vi "Process.vi"(8 "error in":errorcluster, 11 "UI_Scope":refnum<class "UI_Scope.lvclass">) -> (0 "error out":errorcluster, 3 "UI_Scope out":refnum<class "UI_Scope.lvclass">)   [LabVIEW 2016, in "UI_Scope.lvclass"]
doc: "---------------------------------------------------------------\nJKI State Machine Objects™\nhttp://jki.net/state-machine-objects/\nCopyright (C) 2005-2015, JKI <info@jki.net>\nALL RIGHTS RESERVED"
uses:
  UI_Scope.lvclass
  C:/Program Files (x86)/National Instruments/LabVIEW 2016/vi.lib/JKI/JKI SMO/SMO/SMO.lvclass
  <vilib>/JKI/JKI SMO/SMO/Typedefs/Parent Call--Enum.ctl
  <vilib>/JKI/JKI SMO/SMO/SMO.lvclass
panel:
  in  "Close Window":bool
  # "For instructions on how to use the JKI State Machine Objects, examples and video tutorials, visit:\nhttp://jki.net/state-machine-objects/\n\nJKI State Machine Objects™\nhttp://jki.net/state-machine-objects/\nCopyright (C) 2005-2015, JKI <info@jki.net>\nALL RIGHTS RESERVED"
  # "displayScope"
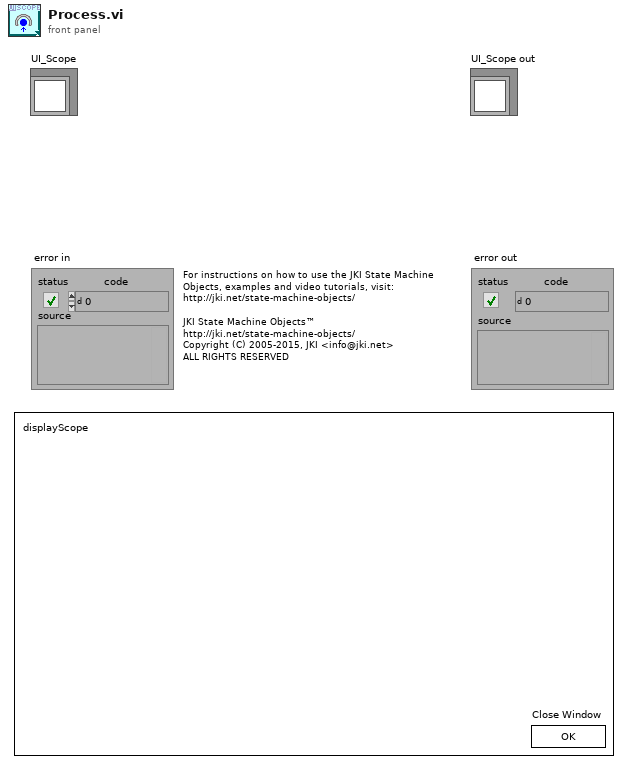
[diagram p1: front panel]
types:
  T1 = typedef "SMO.lvclass/Parent Call--Enum.ctl" = enum16{"Allows parent to run", "Does not request parent to run"}
  T2 = enum32{"invalid app kind", "Development System", "Run Time System", "Student Edition", "Embedded LabVIEW", "Evaluation", "Custom"}
  T3 = enum32{"Invalid", "Standard", "Closed", "Hidden", "Minimized", "Maximized"}
  T4 = enum32{"Bad", "Idle", "Run top level", "Running"}
  T5 = cluster{"Core":cluster{"Current VI Reference":refnum<vi>, "Close Panel on Exit?":bool, "error":errorcluster}, "Self Reference":refnum<class "UI_Scope.lvclass">, "Your string data":string}
  T6 = cluster{"Current VI Reference":refnum<vi>, "Close Panel on Exit?":bool, "error":errorcluster}
  T7 = typedef "SMO.lvclass/Protected Events.ctl" = cluster{"StopProcesses":refnum<user-event>, "AbortProcesses":refnum<user-event>, "Config Changed":refnum<user-event>, "Dependency":refnum<user-event>}
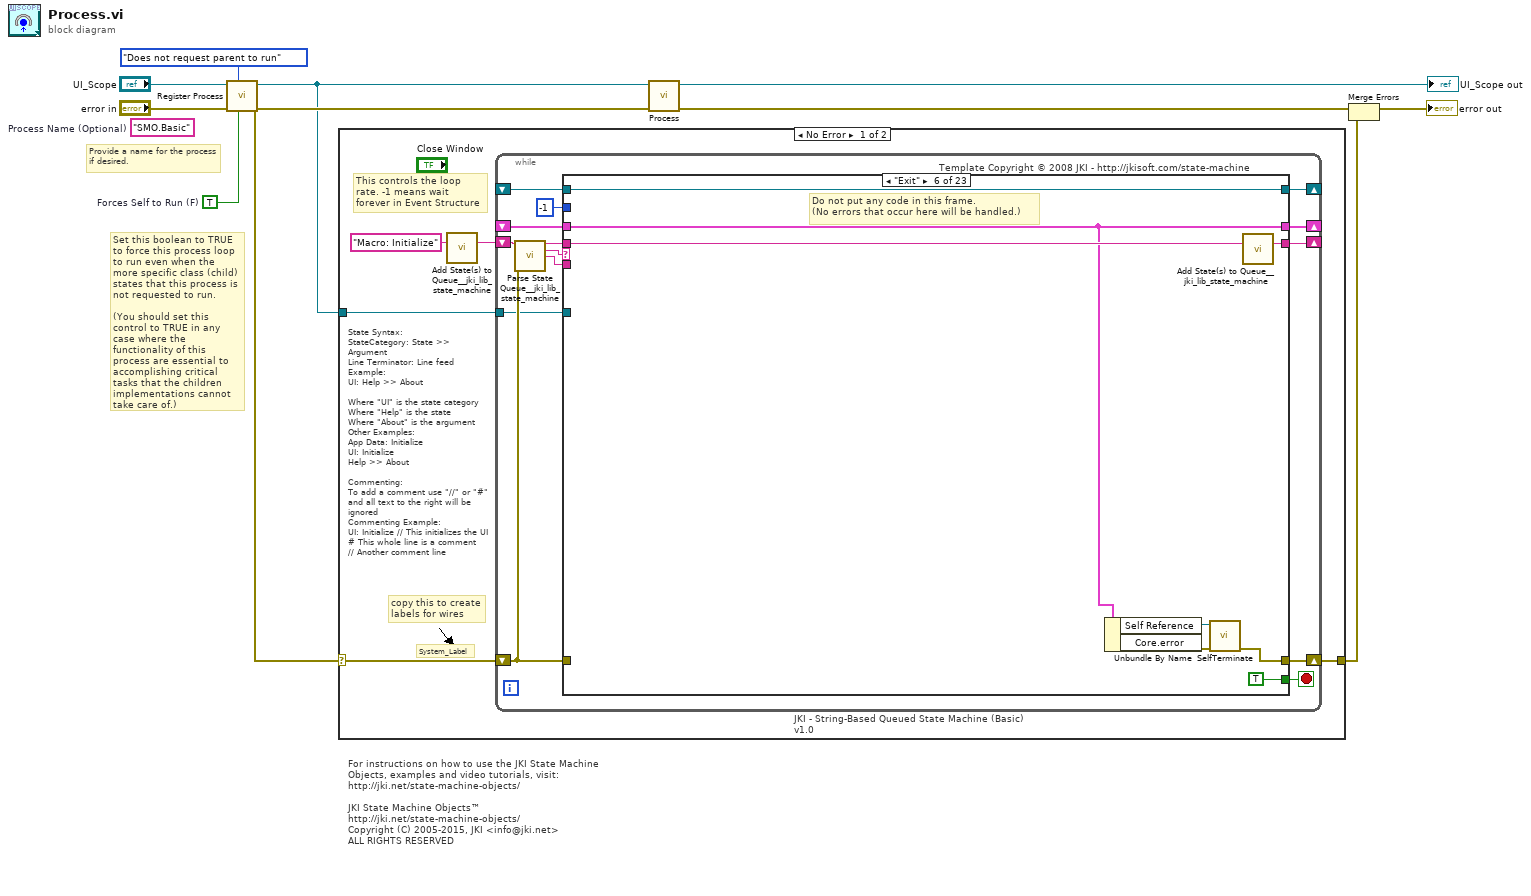
[diagram p0: block diagram]
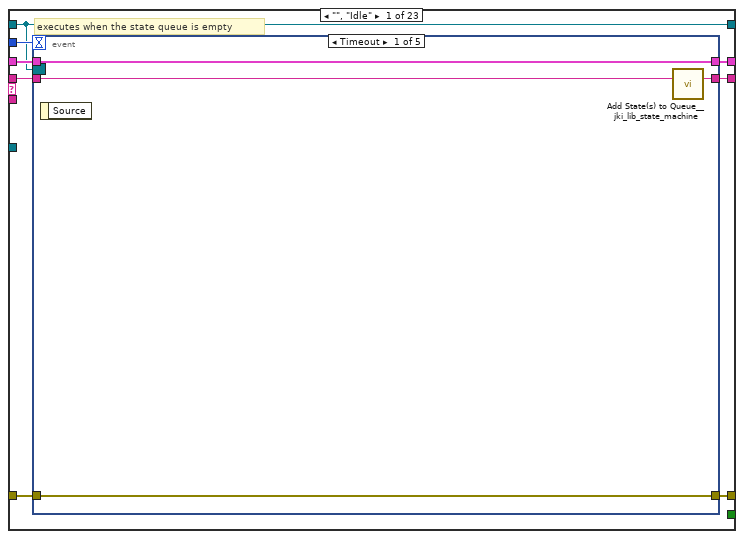
[diagram p2: hidden frame]
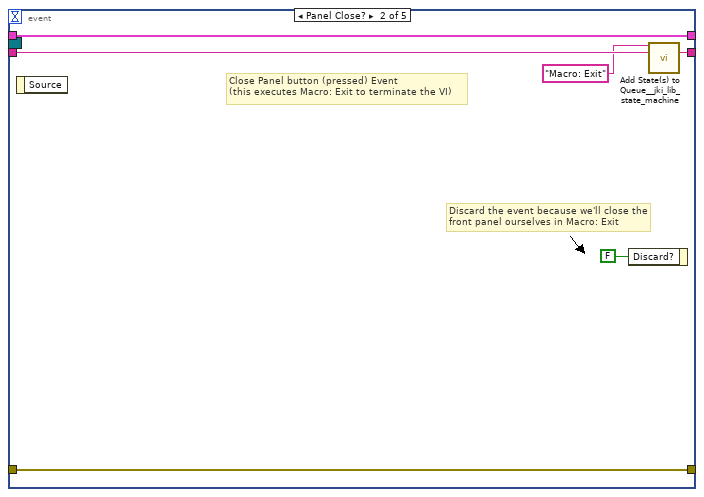
[diagram p3: hidden frame]
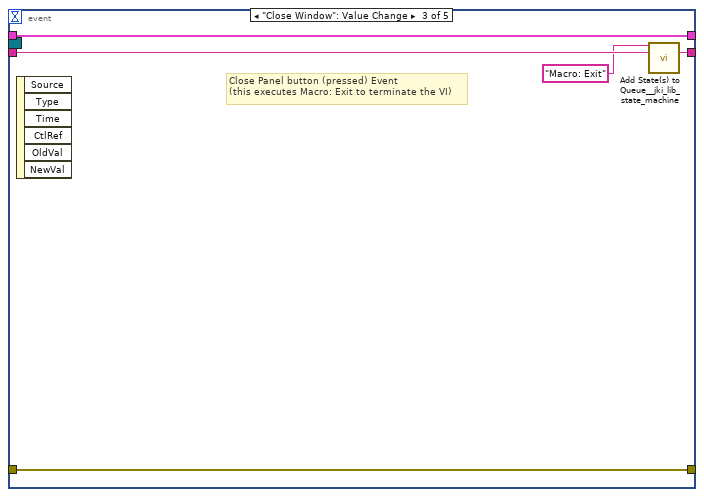
[diagram p4: hidden frame]
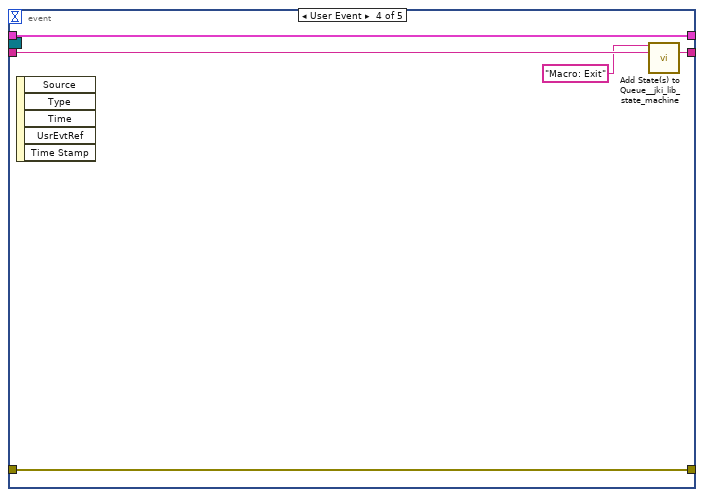
[diagram p5: hidden frame]
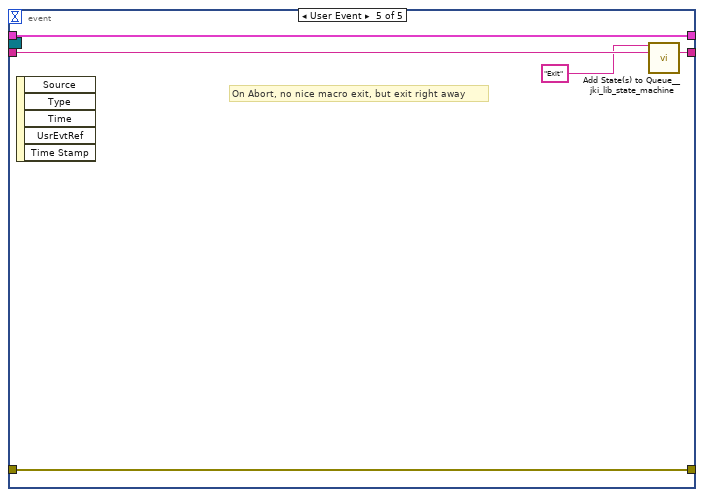
[diagram p6: hidden frame]
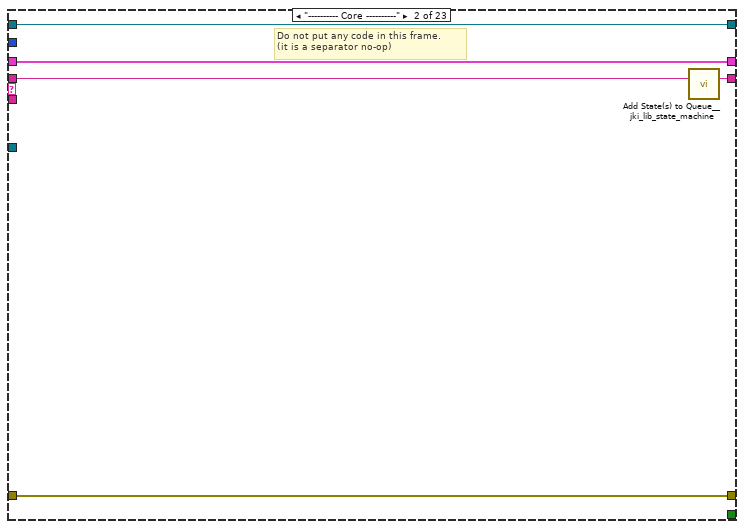
[diagram p7: hidden frame]
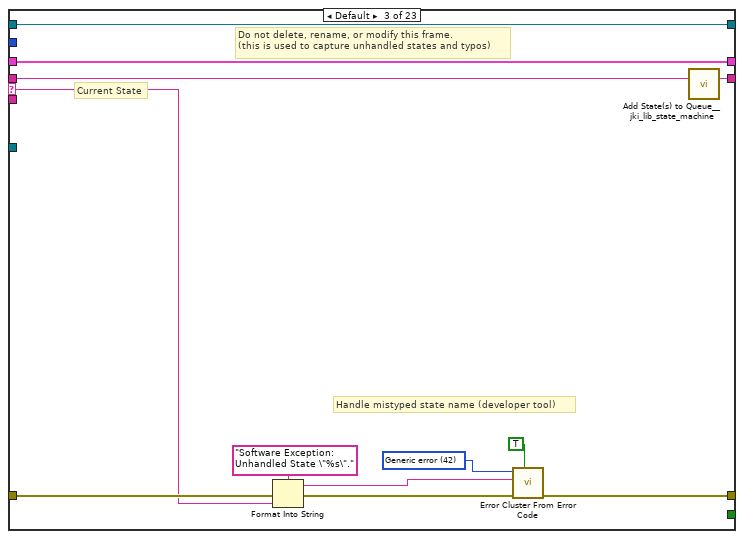
[diagram p8: hidden frame]
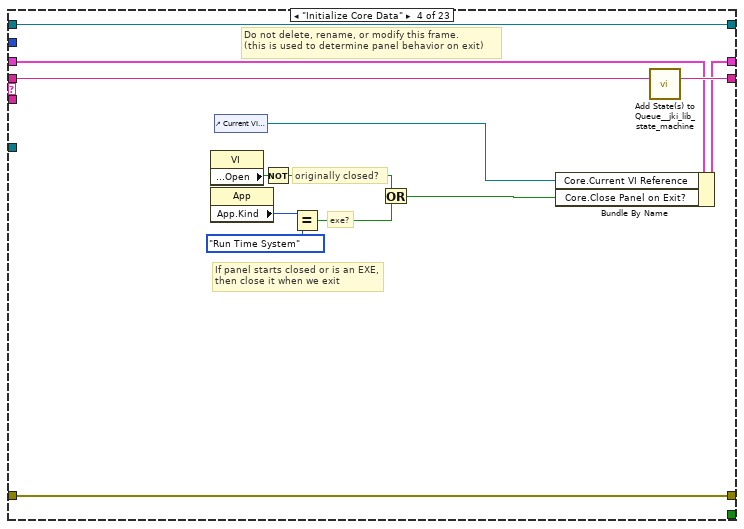
[diagram p9: hidden frame]
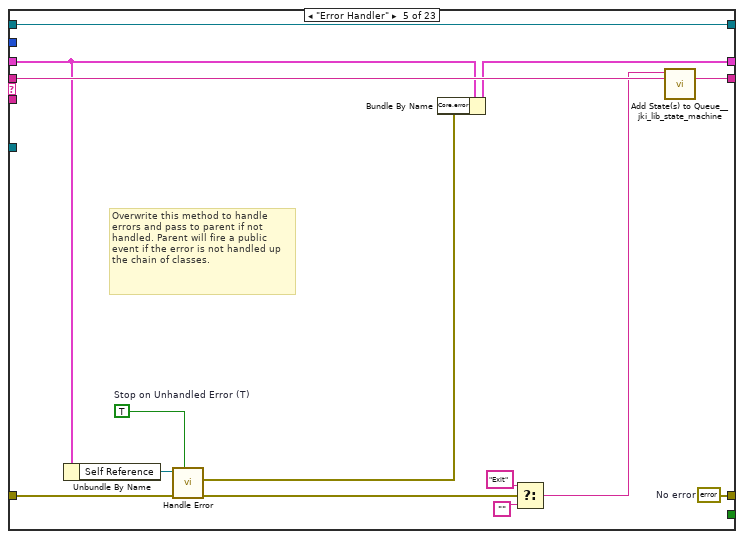
[diagram p10: hidden frame]
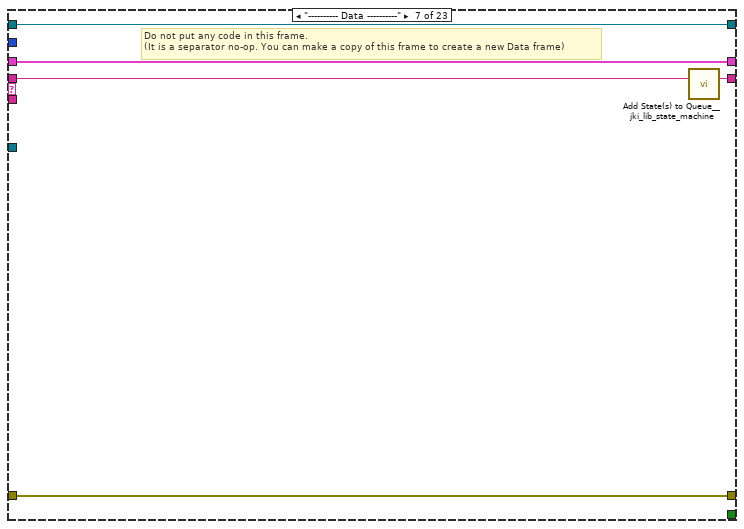
[diagram p11: hidden frame]
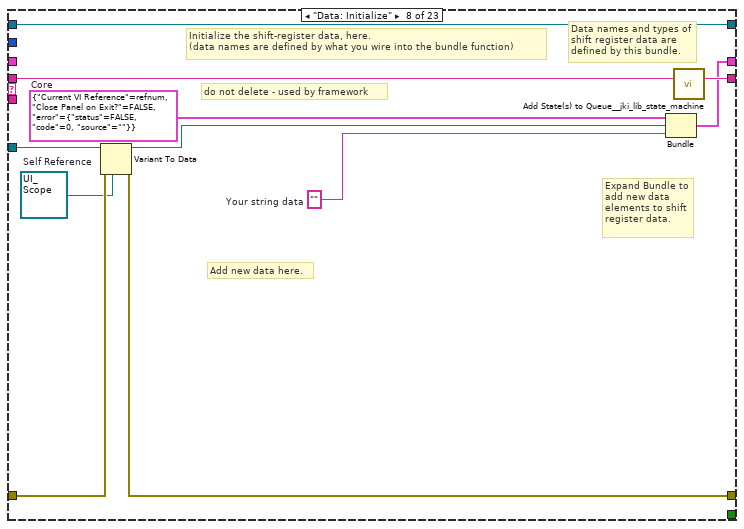
[diagram p12: hidden frame]
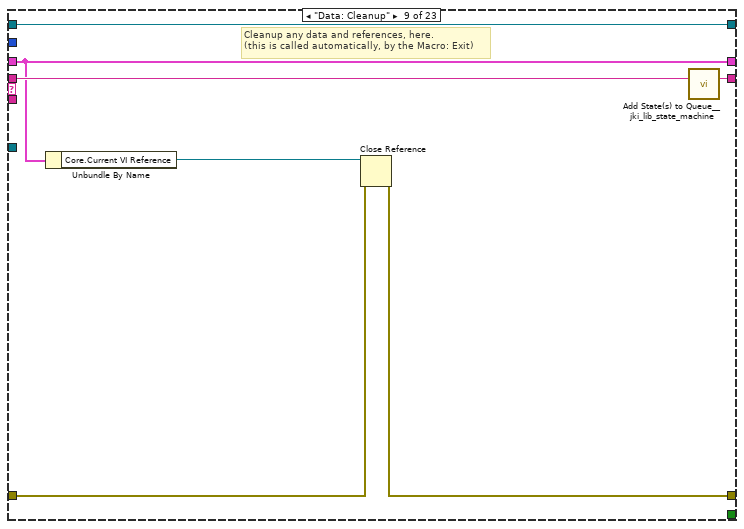
[diagram p13: hidden frame]
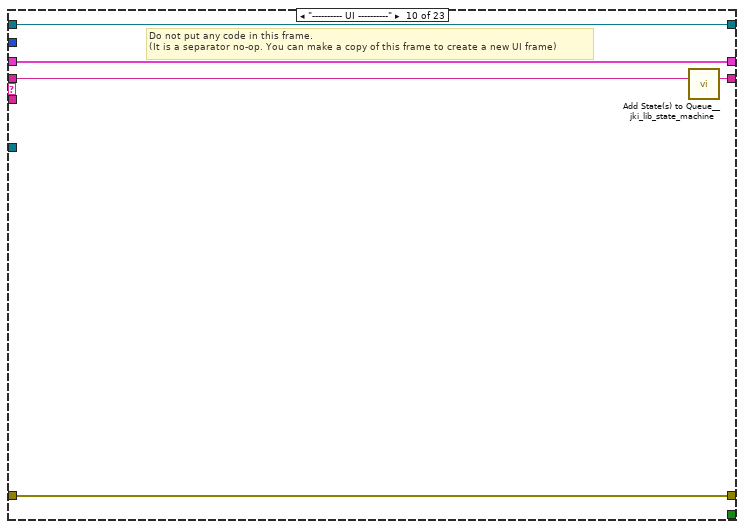
[diagram p14: hidden frame]
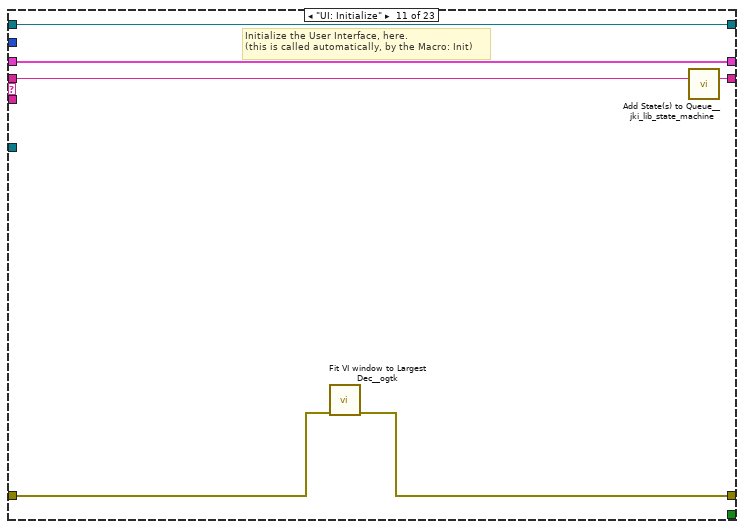
[diagram p15: hidden frame]
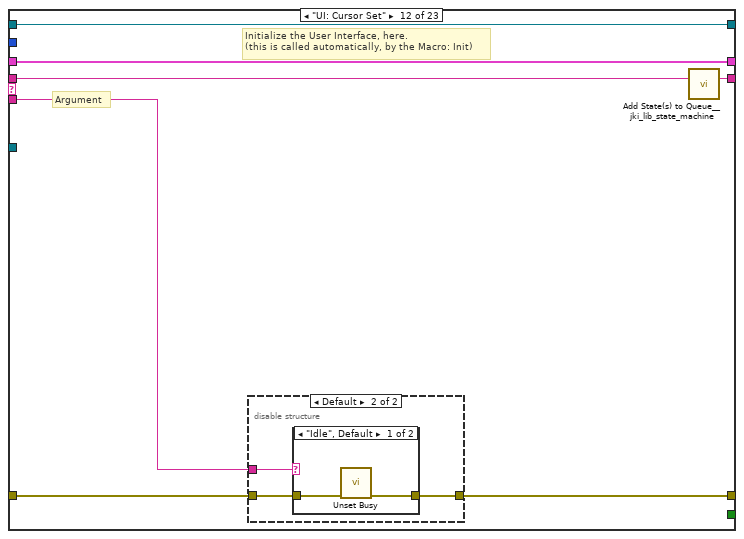
[diagram p16: hidden frame]
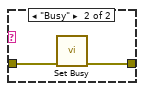
[diagram p18: hidden frame]
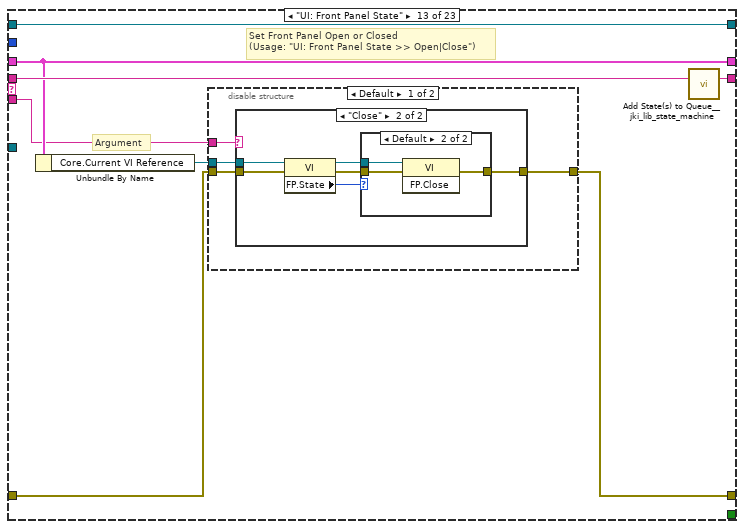
[diagram p19: hidden frame]
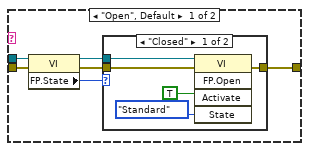
[diagram p20: hidden frame]
diagram:
  w1 = TRUE  # Forces Self to Run (F)
  (unwired) "SMO.Basic"  # Process Name (Optional)
  # "Provide a name for the process\nif desired."
  # "Set this boolean to TRUE to force this process loop to run even when the more specific class (child) states that this process is not requested to run.\n\n(You should set this control to TRUE in any case where the functionality of this process are essential to accomplishing critical tasks that the children implementations cannot take care of.)"
  # "For instructions on how to use the JKI State Machine Objects, examples and video tutorials, visit:\nhttp://jki.net/state-machine-objects/\n\nJKI State Machine Objects™\nhttp://jki.net/state-machine-objects/\nCopyright (C) 2005-2015, JKI <info@jki.net>\nALL RIGHTS RESERVED"
  n1 = call <vilib>:"Register Process.vi"("Forces Self to Run (F)"=w1, "Parent Call"=Parent_Call--Enum."Does not request parent to run", "error in (no error)"="error in", "SMO"="UI_Scope") -> ("error out"=w7:errorcluster, "SMO out"=w6:refnum<class "UI_Scope.lvclass">)  [unwired: 6 in]
  n2 = case shown="No Error" w7 {
    selector: w7 -> [w12 w281]
    tunnel: w6 -> [w13 _]
    tunnel: [w11 w281] -> w3
    frame No Error {
      # "State Syntax:\nStateCategory: State >> Argument\nLine Terminator: Line feed\nExample:\nUI: Help >> About\n\nWhere \"UI\" is the state category\nWhere \"Help\" is the state\nWhere \"About\" is the argument\nOther Examples:\nApp Data: Initialize\nUI: Initialize\nHelp >> About\n\nCommenting:\nTo add a comment use \"//\" or \"#\" and all text to the right will be ignored\nCommenting Example:\nUI: Initialize // This initializes the UI\n# This whole line is a comment\n// Another comment line"
      # "copy this to create labels for wires"
      # "This controls the loop rate. -1 means wait forever in Event Structure"
      # "System_Label"
      n3 = call <vilib>:"Add State(s) to Queue__jki_lib_state_machine.vi"("State(s) in (\"\")"="Macro: Initialize") -> ("States Out"=w15:string)  [unwired: 14 in]
      n4 = while "JKI - String-Based Queued State Machine (Basic) v1.0" {
        shift-right: [w22] -> _
        shift-left: _ -> [w21]
        shift-right: [w25] -> w11
        shift-left: w12 -> [w19]
        shift-right: [w24] -> _
        shift-left: w15 -> [w26]
        tunnel: w13 -> [w18]
        shift-right: [w17] -> _
        shift-left: _ -> [w16]
        stop <- w23 stop-if-true
        # "Template Copyright © 2008 JKI - http://jkisoft.com/state-machine"
        n5 = call <vilib>:"Parse State Queue__jki_lib_state_machine.vi"("State Queue"=w26, "Error In (no error)"=w19) -> ("Remaining States"=w28:string, "Current State"=w29:string, "Arguments"=w27:string)  [unwired: 11 in]
        n6 = case shown="\"Exit\"" w29 {
          selector: w29 -> [_ _ w69 _ _ _ _ _ _ _ _ _ _ _ _ _ _ _ _ _ _ _ _]
          tunnel: w28 -> [w37 w67 w73 w92 w106 w114 w119 w130 w137 w142 w148 w155 w171 w203 w217 w231 w236 w247 w252 w262 w268 w273 w280]
          tunnel: w27 -> [_ _ _ _ _ _ _ _ _ _ _ w149 w165 _ _ _ _ _ _ _ _ _ _]
          tunnel: w21 -> [w35 w64 w71 w83 w100 w107 w116 _ w132 w139 w146 w153 w167 w200 w213 w222 w233 w244 w249 w260 w266 w271 w276]
          tunnel: [w34 w65 w75 w89 w101 w108 w117 w125 w133 w140 w143 w150 w168 w201 w215 w229 w234 w238 w250 w255 w264 w269 w277] -> w25
          tunnel: w19 -> [w33 w65 w74 w89 w102 _ w117 w126 w134 w140 w144 w151 w169 w201 w215 w229 w234 w239 w250 w256 w264 w269 w277]
          tunnel: [w36 w66 w72 w91 w105 w113 w118 w129 w136 w141 w147 w154 w170 w202 w216 w230 w235 w246 w251 w261 w267 w272 w279] -> w24
          tunnel: [_ _ _ _ _ TRUE _ _ _ _ _ _ _ _ _ _ _ _ _ _ _ _ _] -> w23
          tunnel: [w32 w64 w71 w90 w99 w107 w116 w128 w132 w139 w146 w153 w167 w200 w213 w222 w233 w244 w249 w260 w266 w271 w275] -> w22
          tunnel: -1 ("Timeout") -> [w31 _ _ _ _ _ _ _ _ _ _ _ _ _ _ _ _ _ _ _ _ _ _]
          tunnel: w18 -> [_ _ _ _ _ _ _ w123 _ _ _ _ _ _ _ _ _ _ _ _ _ _ _]
          tunnel: [w30 w63 w68 w80 w104 w111 w115 w121 w131 w138 w145 w152 w164 w199 w214 w223 w232 w245 w248 w259 w265 w270 w278] -> w17
          tunnel: w16 -> [w30 w63 w68 w80 w104 w111 w115 w121 w131 w138 w145 w152 w164 w199 w214 w223 w232 w245 w248 _ w265 w270 w278]
          frame "", "Idle" {
            # "executes when the state queue is empty"
            n7 = event shown="[0] Timeout" {
              selector: w30 -> [_ _ _ _ _]
              dyn-events: _ -> [_ _ _ _ _]
              timeout: w31 -> [_ _ _ _ _]
              tunnel: w37 -> [w41 w47 w52 w57 w62]
              tunnel: [w40 w46 w51 w56 w61] -> w36
              tunnel: w35 -> [w39 w44 w49 w54 w59]
              tunnel: [w38 w45 w50 w55 w60] -> w34
              tunnel: w33 -> [w38 w45 w50 w55 w60]
              tunnel: [w39 w44 w49 w54 w59] -> w32
              event Timeout {
                n8 = event-data() -> ()  [unwired: 1 in, 1 out]
                n9 = call <vilib>:"Add State(s) to Queue__jki_lib_state_machine.vi"("State(s) in (\"\")"=w41) -> ("States Out"=w40:string)  [unwired: 14 in]
              }
              event Panel Close? {
                # "Discard the event because we'll close the front panel ourselves in Macro: Exit"
                # "Close Panel button (pressed) Event\n(this executes Macro: Exit to terminate the VI)"
                n10 = event-data() -> ()  [unwired: 1 in, 1 out]
                n11 = event-data("Discard?"=FALSE) -> ()  [unwired: 1 in, 1 out]
                n12 = call <vilib>:"Add State(s) to Queue__jki_lib_state_machine.vi"("State(s) in Front (\"\")"="Macro: Exit", "State(s) in (\"\")"=w47) -> ("States Out"=w46:string)  [unwired: 13 in]
              }
              event "Close Window": Value Change {
                # "Close Panel button (pressed) Event\n(this executes Macro: Exit to terminate the VI)"
                n13 = event-data() -> ()  [unwired: 1 in, 6 out]
                n14 = call <vilib>:"Add State(s) to Queue__jki_lib_state_machine.vi"("State(s) in Front (\"\")"="Macro: Exit", "State(s) in (\"\")"=w52) -> ("States Out"=w51:string)  [unwired: 13 in]
              }
              event User Event {
                n15 = event-data() -> ()  [unwired: 1 in, 5 out]
                n16 = call <vilib>:"Add State(s) to Queue__jki_lib_state_machine.vi"("State(s) in Front (\"\")"="Macro: Exit", "State(s) in (\"\")"=w57) -> ("States Out"=w56:string)  [unwired: 13 in]
              }
              event User Event {
                # "On Abort, no nice macro exit, but exit right away"
                n17 = event-data() -> ()  [unwired: 1 in, 5 out]
                n18 = call <vilib>:"Add State(s) to Queue__jki_lib_state_machine.vi"("State(s) in Front (\"\")"="Exit", "State(s) in (\"\")"=w62) -> ("States Out"=w61:string)  [unwired: 13 in]
              }
            }
          }
          frame "---------- Core ----------" {
            # "Do not put any code in this frame.\n(it is a separator no-op)"
            n19 = call <vilib>:"Add State(s) to Queue__jki_lib_state_machine.vi"("State(s) in (\"\")"=w67) -> ("States Out"=w66:string)  [unwired: 14 in]
          }
          frame Default {
            w78 = 42 items=["No error", "Argument error", "Memory is full", "Out of zone", "End of file", "File already open", "Generic file I/O error", "File not found", "File permission error", "Disk is full", "Duplicate path", "Too many files open", "System feature not enabled", "Resource file not found", "Cannot add resource", "Resource not found", "Image not found", "Image memory error", "Pen does not exist", "Config type invalid", "Config token not found", "Config parse error", "Config memory error", "Bad external code format", "Bad external code offset", "External code not present", "Null window", "Destroy window error", "Null menu", "Print aborted", "Bad print record", "Print driver error", "Windows error during printing", "Memory error during printing", "Print dialog error", "Generic print error", "Invalid device refnum", "Device not found", "Device parameter error", "Device unit error", "Cannot open device", "Device call aborted", "Generic error", "Cancelled by user", "Object ID too low", "Object ID too high", "Object not in heap", "Unknown heap", "Unknown object (invalid DefProc)", "Unknown object (DefProc not in table)", "Message out of range", "Invalid (null) method", "Unknown message", "Manager call not supported", "Bad address", "Network operation in progress", "Network operation timed out", "Connection is busy", "Network attribute not supported", "Network error", "Address in use", "System out of memory", "Connection aborted", "Connection refused", "Not connected", "Already connected", "Connection closed", "Initialization error (interapplication manager)", "Bad occurrence", "Wait on unbound occurrence handler", "Occurrence queue overflow", "Datalog type conflict", "Unused", "Unrecognized type (interapplication manager)", "Memory corrupt", "Failed to make temporary DLL", "Old CIN version", "Drag socket not found", "Failed to load drop-object", "Failed to register OLE object", "Failed to release OLE object", "Format specifier type mismatch", "Unknown format specifier", "Too few format specifiers", "Too many format specifiers", "Scan failed", "Newer CIN version", "Error converting to variant", "Runtime menu error", "Password tampered", "Variant attribute not found", "Incompatible variant data type", "Event data is not available", "Event Store is not present", "Occurrence is not found", "Event Queue is not created", "Event info is not available", "Refnum passed is NULL", "Error retrieving Class GUID", "Error retrieving CoClass GUID", "Error retrieving TypeLib GUID.", "Bad built application magic bytes.", "Specific driver is different from the specific driver associated with the Logical Name.", "There is no session opened to the class driver.", "Max Error", "MAX - Error with config objects", "MAX - Error loading configuration", "MAX - Group not supported"]
            # "Current State"
            # "Do not delete, rename, or modify this frame.\n(this is used to capture unhandled states and typos)"
            # "Handle mistyped state name (developer tool)"
            n20 = Format Into String(format string="Software Exception: Unhandled State \"%s\"." ("message"), error in=w74, w69) -> (resulting string=w77:string, error out=w76:errorcluster)  [unwired: 1 in]
            n21 = call <vilib>:"Error Cluster From Error Code.vi"("show call chain? (False)"=TRUE, "error in (no error)"=w76, "error message (\"\")"=w77, "error code (0)"=w78) -> ("error out"=w75:errorcluster)  [unwired: 5 in]
            n22 = call <vilib>:"Add State(s) to Queue__jki_lib_state_machine.vi"("State(s) in (\"\")"=w73) -> ("States Out"=w72:string)  [unwired: 14 in]
          }
          frame "Initialize Core Data" {
            # "Do not delete, rename, or modify this frame.\n(this is used to determine panel behavior on exit)"
            # "originally closed?"
            # "exe?"
            # "If panel starts closed or is an EXE, then close it when we exit"
            n23 = property class="VI"() -> ("Front Panel.Open"=w88:bool)  [unwired: 2 in, 2 out]
            n24 = property class="App"() -> ("App.Kind"=w87:T2)  [unwired: 2 in, 2 out]
            n25 = control-ref of="Current VI Reference"() -> (w81:refnum<vi>)
            n26 = Not(x=w88) -> (.not. x?=w85:bool)
            n27 = Equal?(x=w87, y=T2."Run Time System" ("Application:Kind")) -> (x = y?=w84:bool)
            n28 = Or(x=w85, y=w84) -> (x .or. y?=w82:bool)
            n29 = Bundle By Name(cluster=w83, "Core.Current VI Reference"=w81, "Core.Close Panel on Exit?"=w82) -> (w90:T5)
            n30 = call <vilib>:"Add State(s) to Queue__jki_lib_state_machine.vi"("State(s) in (\"\")"=w92) -> ("States Out"=w91:string)  [unwired: 14 in]
          }
          frame "Error Handler" {
            w93 = TRUE  # Stop on Unhandled Error (T)
            w101 = errorcluster {"status"=FALSE, "code"=0, "source"=""}  # No error
            # "Overwrite this method to handle errors and pass to parent if not handled. Parent will fire a public event if the error is not handled up the chain of classes."
            n31 = Unbundle By Name(w100) -> ("Self Reference"=w103:refnum<class "UI_Scope.lvclass">)
            n32 = call-dynamic "Handle Error.vi"("Stop on Unhandled Error (T)"=w93, "error in"=w102, "SMO"=w103) -> ("handling error"=w94:errorcluster, "Unhandled error"=w97:errorcluster)  [unwired: 6 in, 1 out]
            n33 = Bundle By Name(cluster=w100, "Core.error"=w97) -> (w99:T5)
            n34 = Select(t="Exit", s=w94, f="") -> (s? t:f=w98:string)
            n35 = call <vilib>:"Add State(s) to Queue__jki_lib_state_machine.vi"("State(s) in Front (\"\")"=w98, "State(s) in (\"\")"=w106) -> ("States Out"=w105:string)  [unwired: 13 in]
          }
          frame "Exit" {
            # "Do not put any code in this frame.\n(No errors that occur here will be handled.)"
            n36 = Unbundle By Name(w107) -> ("Self Reference"=w109:refnum<class "UI_Scope.lvclass">, "Core.error"=w110:errorcluster)
            n37 = call <vilib>:"SelfTerminate.vi"("error in (no error)"=w110, "SMO in"=w109) -> ("error out"=w108:errorcluster)  [unwired: 8 in, 1 out]
            n38 = call <vilib>:"Add State(s) to Queue__jki_lib_state_machine.vi"("State(s) in (\"\")"=w114) -> ("States Out"=w113:string)  [unwired: 14 in]
          }
          frame "---------- Data ----------" {
            # "Do not put any code in this frame.\n(It is a separator no-op. You can make a copy of this frame to create a new Data frame)"
            n39 = call <vilib>:"Add State(s) to Queue__jki_lib_state_machine.vi"("State(s) in (\"\")"=w119) -> ("States Out"=w118:string)  [unwired: 14 in]
          }
          frame "Data: Initialize" {
            w120 = T6 {"Current VI Reference"=refnum, "Close Panel on Exit?"=FALSE, "error"={"status"=FALSE, "code"=0, "source"=""}}  # Core
            w124 = refnum<class "UI_Scope.lvclass"> refnum  # Self Reference
            w127 = ""  # Your string data
            # "do not delete - used by framework"
            # "Expand Bundle to add new data elements to shift register data."
            # "Add new data here."
            # "Data names and types of shift register data are defined by this bundle."
            # "Initialize the shift-register data, here.\n(data names are defined by what you wire into the bundle function)"
            n40 = Variant To Data(error in=w126, type=w124, Variant=w123) -> (data=w122:refnum<class "UI_Scope.lvclass">, error out=w125:errorcluster)
            n41 = Bundle("Core"=w120, "Self Reference"=w122, "Your string data"=w127) -> (w128:T5)  [unwired: 1 in]
            n42 = call <vilib>:"Add State(s) to Queue__jki_lib_state_machine.vi"("State(s) in (\"\")"=w130) -> ("States Out"=w129:string)  [unwired: 14 in]
          }
          frame "Data: Cleanup" {
            # "Cleanup any data and references, here.\n(this is called automatically, by the Macro: Exit)"
            n43 = Unbundle By Name(w132) -> ("Core.Current VI Reference"=w135:refnum<vi>)
            n44 = Close Reference(reference=w135, error in (no error)=w134) -> (error out=w133:errorcluster)
            n45 = call <vilib>:"Add State(s) to Queue__jki_lib_state_machine.vi"("State(s) in (\"\")"=w137) -> ("States Out"=w136:string)  [unwired: 14 in]
          }
          frame "---------- UI ----------" {
            # "Do not put any code in this frame.\n(It is a separator no-op. You can make a copy of this frame to create a new UI frame)"
            n46 = call <vilib>:"Add State(s) to Queue__jki_lib_state_machine.vi"("State(s) in (\"\")"=w142) -> ("States Out"=w141:string)  [unwired: 14 in]
          }
          frame "UI: Initialize" {
            # "Initialize the User Interface, here.\n(this is called automatically, by the Macro: Init)"
            n47 = call <userlib>:"Fit VI window to Largest Dec__ogtk.vi"("error in (no error)"=w144) -> ("error out"=w143:errorcluster)  [unwired: 5 in, 1 out]
            n48 = call <vilib>:"Add State(s) to Queue__jki_lib_state_machine.vi"("State(s) in (\"\")"=w148) -> ("States Out"=w147:string)  [unwired: 14 in]
          }
          frame "UI: Cursor Set" {
            # "Argument"
            # "Initialize the User Interface, here.\n(this is called automatically, by the Macro: Init)"
            n49 = disable-structure shown="Default" {
              disable-tunnel: w151 -> [w156 w159]
              disable-tunnel: [w156 w158] -> w150
              disable-tunnel: w149 -> [_ w157]
              frame condition #0 {
              }
              frame condition #1 (active) {
                n50 = case shown="\"Idle\", Default" w157 {
                  tunnel: w159 -> [w161 w163]
                  tunnel: [w160 w162] -> w158
                  frame "Idle", Default {
                    n51 = call <vilib>:"Unset Busy.vi"("error in (no error)"=w161) -> ("error out"=w160:errorcluster)  [unwired: 10 in]
                  }
                  frame "Busy" {
                    n52 = call <vilib>:"Set Busy.vi"("error in (no error)"=w163) -> ("error out"=w162:errorcluster)  [unwired: 9 in, 1 out]
                  }
                }
              }
            }
            n53 = call <vilib>:"Add State(s) to Queue__jki_lib_state_machine.vi"("State(s) in (\"\")"=w155) -> ("States Out"=w154:string)  [unwired: 14 in]
          }
          frame "UI: Front Panel State" {
            # "Argument"
            # "Set Front Panel Open or Closed\n(Usage: \"UI: Front Panel State >> Open|Close\")"
            n54 = Unbundle By Name(w167) -> ("Core.Current VI Reference"=w166:refnum<vi>)
            n55 = disable-structure shown="Default" {
              disable-tunnel: w169 -> [w175 w198]
              disable-tunnel: [w174 w198] -> w168
              disable-tunnel: w166 -> [w173 _]
              disable-tunnel: w165 -> [w172 _]
              frame condition #0 (active) {
                n56 = case shown="\"Close\"" w172 {
                  tunnel: w175 -> [w179 w192]
                  tunnel: [w181 w193] -> w174
                  tunnel: w173 -> [w180 w190]
                  frame "Open", Default {
                    n57 = property class="VI"(reference=w180, error in=w179) -> (reference out=w177:refnum<vi>, error out=w178:errorcluster, "FP.State"=w176:T3)
                    n58 = case shown="\"Closed\"" w176 {
                      tunnel: [w184 w187] -> w181
                      tunnel: w178 -> [w183 w187]
                      tunnel: w177 -> [w182 _]
                      frame "Closed" {
                        n59 = invoke class="VI" method="FP.Open"(reference=w182, error in=w183, "Activate"=TRUE, "State"=T3."Standard") -> (error out=w184:errorcluster)  [unwired: 1 in, 4 out]
                      }
                      frame Default {
                      }
                    }
                  }
                  frame "Close" {
                    n60 = property class="VI"(reference=w190, error in=w192) -> (reference out=w189:refnum<vi>, error out=w191:errorcluster, "FP.State"=w188:T3)
                    n61 = case shown="Default" w188 {
                      tunnel: [w194 w197] -> w193
                      tunnel: w191 -> [w194 w196]
                      tunnel: w189 -> [_ w195]
                      frame "Invalid", "Closed" {
                      }
                      frame Default {
                        n62 = invoke class="VI" method="FP.Close"(reference=w195, error in=w196) -> (error out=w197:errorcluster)  [unwired: 1 in, 2 out]
                      }
                    }
                  }
                }
              }
              frame condition #1 {
              }
            }
            n63 = call <vilib>:"Add State(s) to Queue__jki_lib_state_machine.vi"("State(s) in (\"\")"=w171) -> ("States Out"=w170:string)  [unwired: 14 in]
          }
          frame "---------- Macro ----------" {
            # "Do not put any code in this frame.\n(It is a separator no-op. You can make a copy of this frame to create a new Macro frame)"
            n64 = call <vilib>:"Add State(s) to Queue__jki_lib_state_machine.vi"("State(s) in (\"\")"=w203) -> ("States Out"=w202:string)  [unwired: 14 in]
          }
          frame "Macro: Initialize" {
            w208 = "UI: Initialize\nUI: Front Panel State >> Open"  # UI: Initialize UI: Front Panel State >> Open
            w204 = "Process: Sync"
            # "Initialization Macro\n(This is called once, when the VI starts)"
            n65 = control-ref of="This VI"() -> (w206:refnum<vi>)
            n66 = property class="VI"(reference=w206) -> ("Exec.State"=w205:T4)  [unwired: 1 in, 2 out]
            n67 = Equal?(x=w205, y=T4."Run top level") -> (x = y?=w211:bool)
            n68 = Select(t=w204, s=w211, f="") -> ()  [unwired: 1 out]
            n69 = call <vilib>:"Add State(s) to Queue__jki_lib_state_machine.vi"("State(s) in Front (\"\")"="Data: Initialize\nInitialize Core Data\nEvents: Register", "State(s) in (\"\")"=w204, "State(s) at Back (\"\")"=w208) -> ("States Out"=w207:string)  [unwired: 12 in]
            n70 = call <vilib>:"Add State(s) to Queue__jki_lib_state_machine.vi"("State(s) in Front (\"\")"=w207, "State(s) in (\"\")"=w217) -> ("States Out"=w216:string)  [unwired: 13 in]
          }
          frame "Macro: Exit" {
            # "Exit Macro\n(This is called once, when the VI exits)"
            n71 = Unbundle By Name(w222) -> ("Core.Close Panel on Exit?"=w228:bool)
            n72 = Select(t="UI: Front Panel State >> Close", s=w228, f="") -> (s? t:f=w225:string)
            n73 = call <vilib>:"Add State(s) to Queue__jki_lib_state_machine.vi"("State(s) in Front (\"\")"="Data: Cleanup\nEvents: Unregister", "State(s) in (\"\")"="Process: Sync", "State(s) at Back (\"\")"="Exit") -> ("States Out"=w219:string)  [unwired: 12 in]
            n74 = call <vilib>:"Add State(s) to Queue__jki_lib_state_machine.vi"("State(s) in (\"\")"=w225, "State(s) at Back (\"\")"=w219) -> ("States Out"=w224:string)  [unwired: 13 in]
            n75 = call <vilib>:"Add State(s) to Queue__jki_lib_state_machine.vi"("State(s) in Front (\"\")"=w224, "State(s) in (\"\")"=w231) -> ("States Out"=w230:string)  [unwired: 13 in]
          }
          frame "---------- Process ----------" {
            # "Template Separator\n(You can make a copy of, or modify, this frame)"
            n76 = call <vilib>:"Add State(s) to Queue__jki_lib_state_machine.vi"("State(s) in (\"\")"=w236) -> ("States Out"=w235:string)  [unwired: 14 in]
          }
          frame "Process: Sync" {
            n77 = Unbundle By Name(w244) -> ("Self Reference"=w240:refnum<class "UI_Scope.lvclass">)
            n78 = call <vilib>:"WaitOnProcessSync.vi"("error in (no error)"=w239, "SMO"=w240) -> ("error out"=w238:errorcluster, "Don't run?"=w243:bool)  [unwired: 7 in, 1 out]
            n79 = Select(t="Data: Cleanup\nEvents: Unregister\nExit", s=w243, f="") -> (s? t:f=w237:string)
            n80 = call <vilib>:"Add State(s) to Queue__jki_lib_state_machine.vi"("State(s) in Front (\"\")"=w237, "State(s) in (\"\")"=w247) -> ("States Out"=w246:string)  [unwired: 13 in]
          }
          frame "---------- Events ----------" {
            # "Template Separator\n(You can make a copy of, or modify, this frame)"
            n81 = call <vilib>:"Add State(s) to Queue__jki_lib_state_machine.vi"("State(s) in (\"\")"=w252) -> ("States Out"=w251:string)  [unwired: 14 in]
          }
          frame "Events: Register" {
            # "Expand to add\nmore events"
            n82 = Unbundle By Name(w260) -> ("Self Reference"=w257:refnum<class "UI_Scope.lvclass">)
            n83 = call <vilib>:"GetProtectedEvents.vi"("SMO"=w257) -> ("error out"=w253:errorcluster, "SMO Protected Events"=w258:T7)  [unwired: 8 in, 1 out]
            n84 = register-events(w258) -> (reference out=w259:refnum<event-registration>, error out=w254:errorcluster)  [unwired: 2 in]
            n85 = Merge Errors(w256, w254, w253) -> (w255:errorcluster)
            n86 = call <vilib>:"Add State(s) to Queue__jki_lib_state_machine.vi"("State(s) in (\"\")"=w262) -> ("States Out"=w261:string)  [unwired: 14 in]
          }
          frame "Events: Unregister" {
            n87 = Unregister For Events(event registration refnum=w265, error in=w264) -> (error out=w263:errorcluster)
            n88 = call <vilib>:"Clear Errors.vi"("error in (no error)"=w263) -> ()  [unwired: 5 in, 2 out]
            n89 = call <vilib>:"Add State(s) to Queue__jki_lib_state_machine.vi"("State(s) in (\"\")"=w268) -> ("States Out"=w267:string)  [unwired: 14 in]
          }
          frame "---------- Action ----------" {
            n90 = call <vilib>:"Add State(s) to Queue__jki_lib_state_machine.vi"("State(s) in (\"\")"=w273) -> ("States Out"=w272:string)  [unwired: 14 in]
          }
          frame "Action: Template" {
            n91 = Unbundle By Name(w276) -> ("Self Reference"=w274:refnum<class "UI_Scope.lvclass">)
            n92 = Bundle By Name(cluster=w276, "Self Reference"=w274) -> (w275:T5)
            n93 = call <vilib>:"Add State(s) to Queue__jki_lib_state_machine.vi"("State(s) in (\"\")"=w280) -> ("States Out"=w279:string)  [unwired: 14 in]
          }
        }
      }
    }
    frame Error {
    }
  }
  n94 = call-parent "Process.vi"("error in"=w7, "SMO"=w6) -> ("error out"=w4:errorcluster, "SMO out"=→"UI_Scope out":refnum<class "UI_Scope.lvclass">)  [unwired: 8 in]
  n95 = Merge Errors(w4, w3) -> (→"error out":errorcluster)
